vi "Signal processing testing.vi"() -> ()   [LabVIEW 2020]
doc: "This example demonstrates how to read N channels of analog input from a LINX device."
uses:
  <vilib>/MakerHub/LINX/Public/Peripherals/Analog/Analog Read N Chans.vi
  <vilib>/MakerHub/LINX/Private/Local IO/LinxAnalogRead.vi
  <vilib>/MakerHub/LINX/Public/Utilities/Check Channel.vi
  <vilib>/MakerHub/LINX/Public/Utilities/Open Serial.vi
  <vilib>/MakerHub/LINX/Private/Utilties/Generate Error.vi
  <vilib>/Analysis/Matrix/Numeric/Conversions/Array To Matrix - RA.vi
  <vilib>/Utility/file.llb/Write Delimited Spreadsheet (DBL).vi
  <vilib>/MakerHub/LINX/LMH-LINX.lvlib
  <vilib>/Analysis/Matrix/NI_Matrix.lvlib
panel:
  in  "B 6":dbl
  in  "A 6":dbl
  out "Weight":dbl
  out "Voltage 3":dbl
  in  "Analog Port 6":dbl
  in  "B 5":dbl
  in  "A 5":dbl
  out "Pressure (PSI) 2":dbl
  out "Voltage 2":dbl
  in  "Analog Port 5":dbl
  in  "Input pressure (PSI)":dbl
  in  "B 4":dbl
  in  "A 4":dbl
  out "Pressure (PSI)":dbl
  out "Voltage":dbl
  in  "Analog Port 4":dbl
  in  "C 3":dbl
  in  "B 3":dbl
  in  "A 3":dbl
  out "Temperature (F) 3":dbl
  out "Temperature (C) 3":dbl
  out "Temperature (K) 3":dbl
  out "Resistance 3":dbl
  in  "Analog Port 3":dbl
  in  "C 2":dbl
  in  "B 2":dbl
  in  "A 2":dbl
  out "Temperature (F) 2":dbl
  out "Temperature (C) 2":dbl
  out "Temperature (K) 2":dbl
  out "Resistance 2":dbl
  in  "Analog Port 2":dbl
  in  "Input temp (C)":dbl
  in  "C":dbl
  in  "B":dbl
  in  "A":dbl
  out "Temperature (F)":dbl
  out "Temperature (C)":dbl
  out "Temperature (K)":dbl
  out "WRITING TO FILE":bool
  in  "?":bool
  out "error out":errorcluster
  out "Full filepath":string
  in  "Path":path
  in  "File extension":string
  in  "Filename":string
  out "Resistance":dbl
  in  "Analog Port":dbl
  out "Time Stamp":timestamp
  out "PT1 reading":dbl(graph)
  in  "Stop Button":bool
  out "Loop Rate (Hz)":u32
  in  "Serial Port":refnum<visa-resource-name>
  # "Thermistor Calibration Program\nThis program gathers data points necessary to calibrate an NTC 10K Thermistor.\n It also allows for the testing of found A, B, and C values via user input."
  # "TM1"
  # "PT1"
  # "TM2"
  # "TM3"
  # "PT2"
  # "LC1"
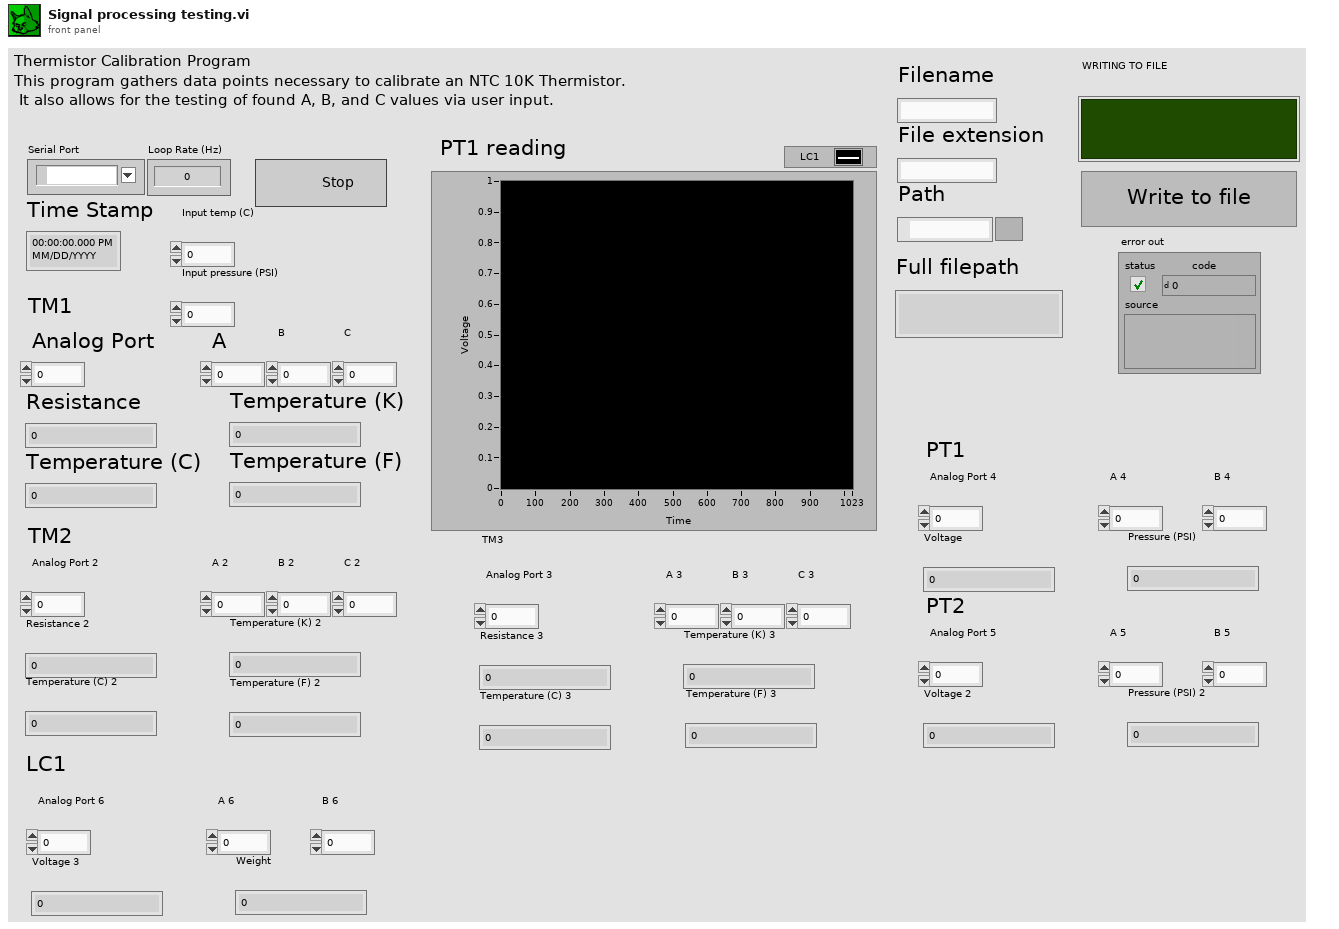
[diagram p1: front panel]
types:
  T1 = typedef "LMH-LINX.lvlib/LINX Ref.ctl" = cluster{"IO":T2, "Interface":T3, "LINX Device Config":T4}
  T2 = typedef "LMH-LINX.lvlib/Platform.ctl" = enum16{"Remote", "Local"}
  T3 = typedef "LMH-LINX.lvlib/Interface.ctl" = enum16{"Serial", "TCP"}
  T4 = typedef "LMH-LINX.lvlib/Device.lvlib/LINX Device Config.ctl" = cluster{"Interface":T3, "COM Port":refnum<visa-resource-name>, "TCP Configuration":T5, "Device Family":u8, "Device ID":u8, "Device Name":string, "TCP Ref":refnum<k5>, "Channels":T6}
  T5 = typedef "LMH-LINX.lvlib/Device.lvlib/TCP Config.ctl" = cluster{"IP Address":string, "Port":u16}
  T6 = typedef "LMH-LINX.lvlib/Channels.ctl" = cluster{"DI":u8[], "DO":u8[], "AI":u8[], "AO":u8[], "PWM":u8[], "QE":u8[], "UART":u8[], "I2C 2":u8[], "SPI":u8[], "CAN":u8[], "Servo":u8[], "AI Ref (V)":dbl, "AI Resolution (Bits)":u8, "AO Ref (V)":dbl, "AO Resolution (Bits)":u8}
  T7 = typedef "NI_Matrix.lvlib/RealMatrix.ctl" = dbl[][]
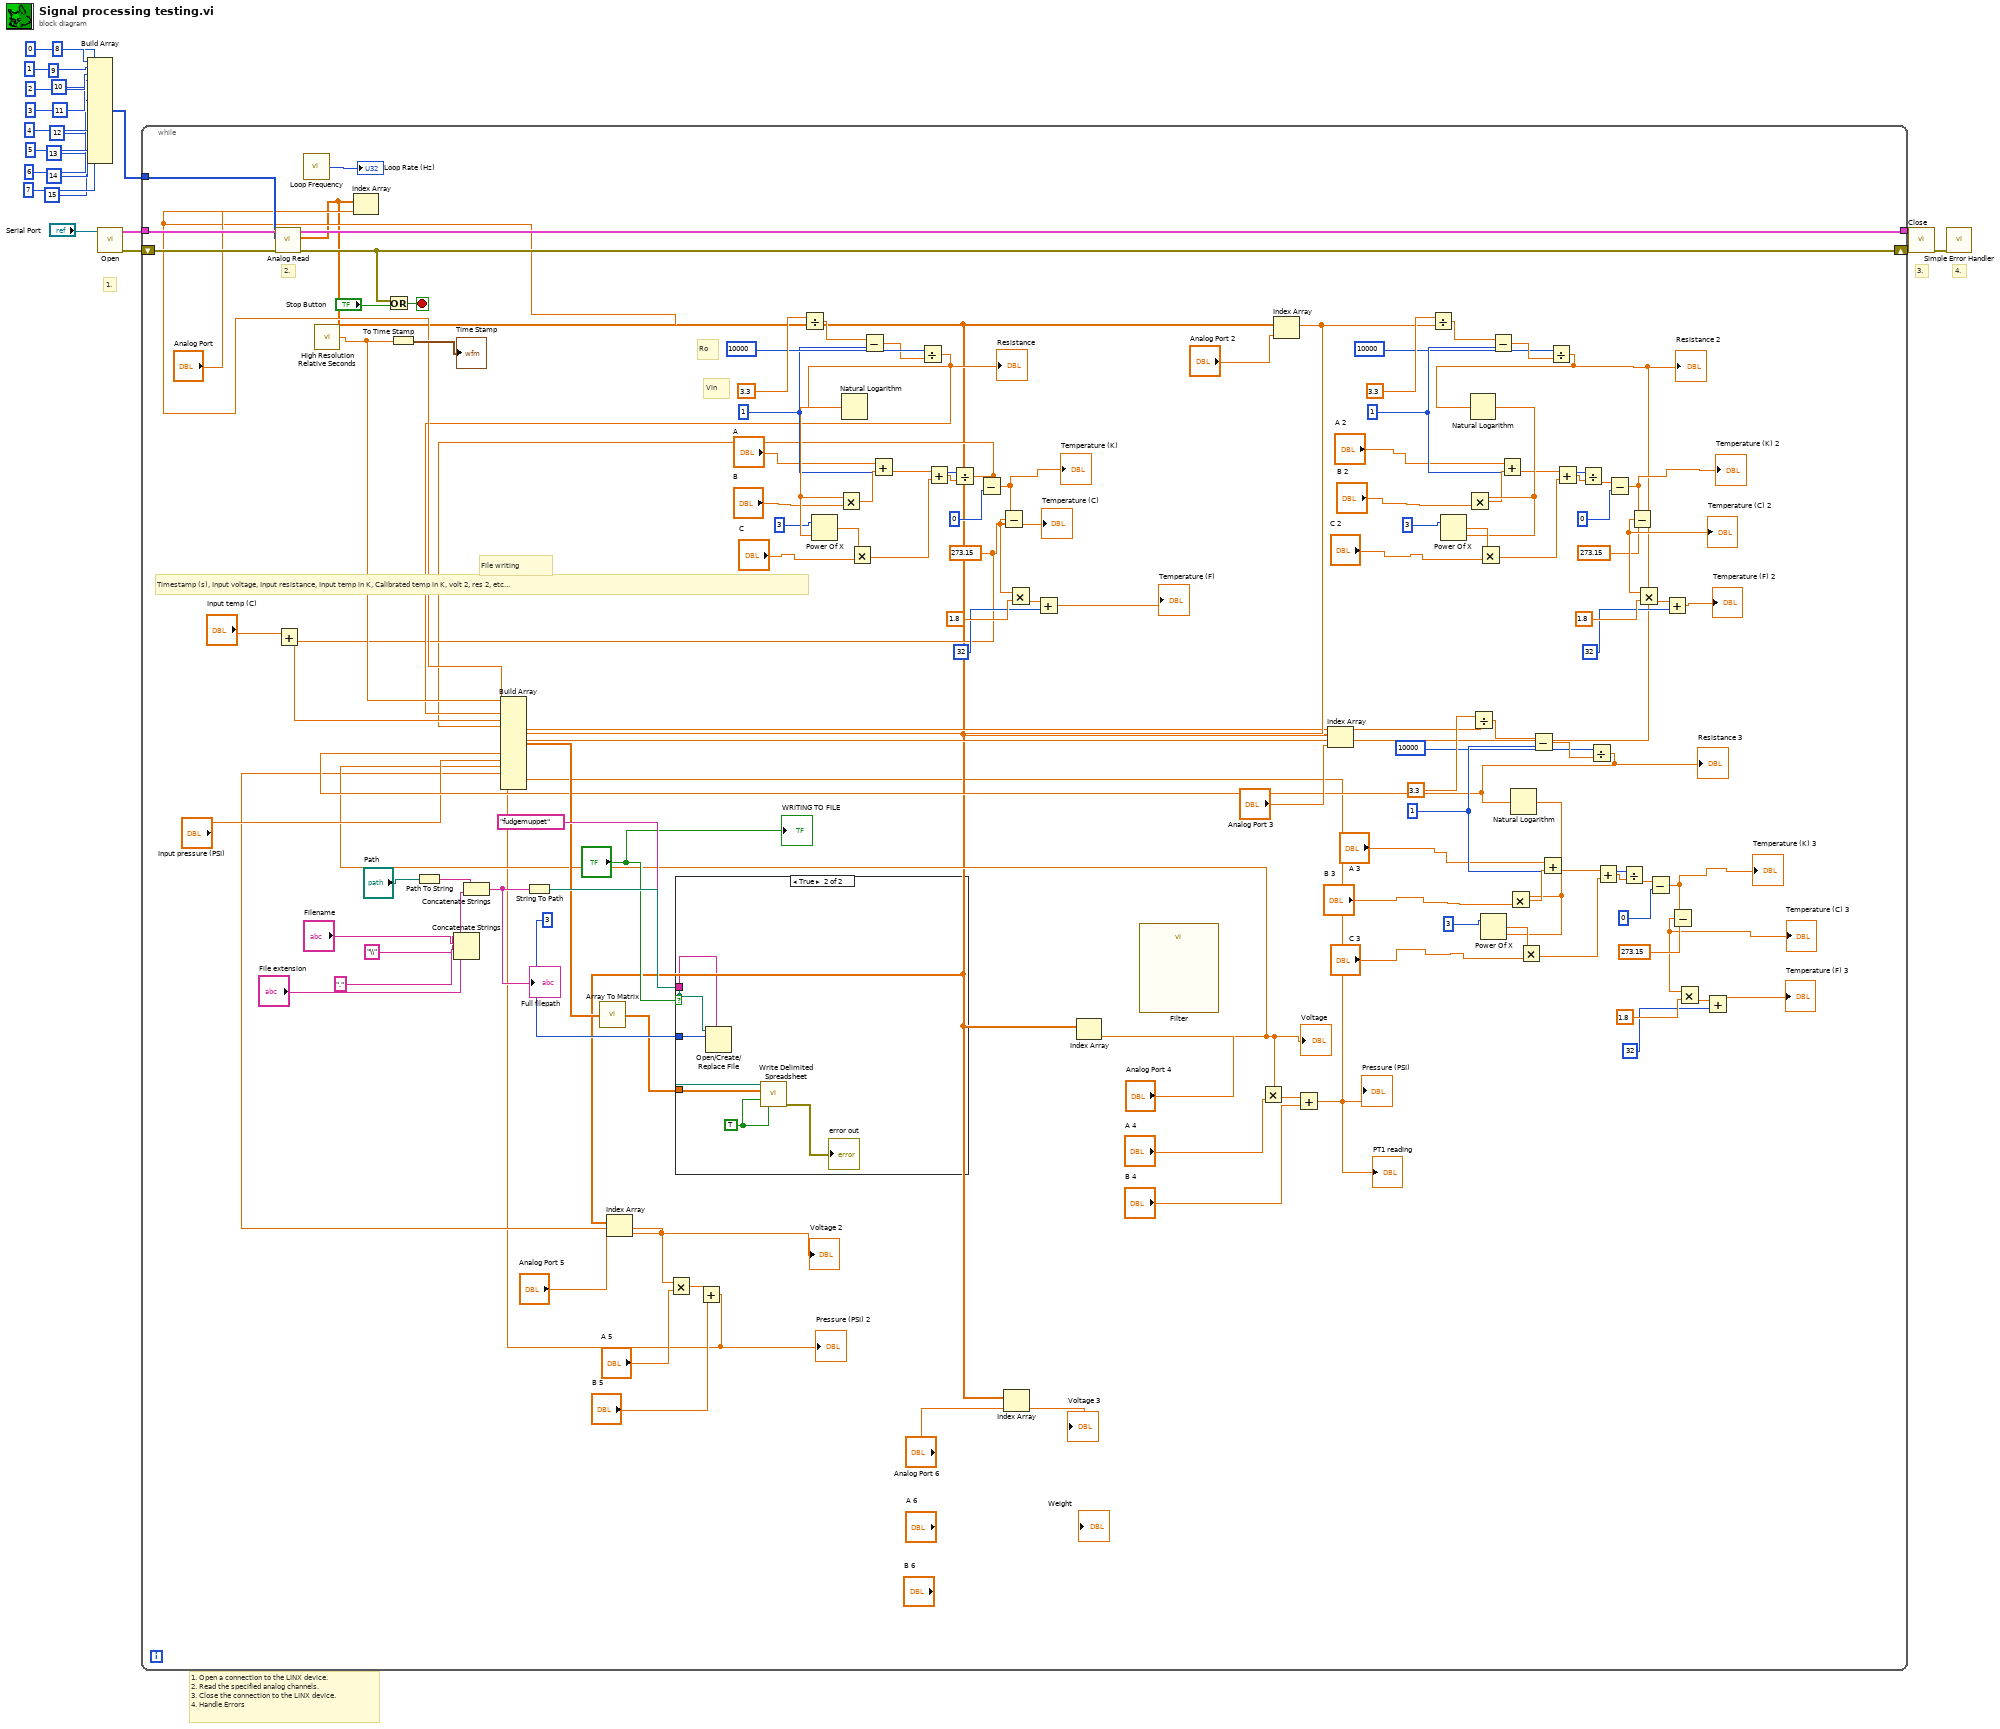
[diagram p0: block diagram]
diagram:
  # "1. Open a connection to the LINX device.\n2. Read the specified analog channels.\n3. Close the connection to the LINX device.\n4. Handle Errors"
  # "4."
  # "3."
  # "1."
  n1 = Build Array(0, 1, 2, 3, 4, 5, 6, 7, 8, 9, 10, 11, 12, 13, 14, 15) -> (w17:i32[])
  n2 = call-poly <vilib>:"Open.vi"("Serial Port"="Serial Port") -> ("Error Out"=w22:errorcluster, "LINX Resource"=w23:T1)  [unwired: 8 in, 1 out]
  n3 = while {
    tunnel: w23 -> [w146]
    tunnel: [w144] -> w21
    shift-right: [w141] -> w20
    shift-left: w22 -> [w145]
    tunnel: w17 -> [w140]
    stop <- w143 stop-if-true
    w61 = 1
    w84 = 1
    w100 = 273.15
    w109 = 1
    # "Timestamp (s), Input voltage, Input resistance, Input temp in K, Calibrated temp in K, volt 2, res 2, etc..."
    # "File writing"
    # "Vin"
    # "Ro"
    # "2."
    n4 = call-poly <vilib>:"Analog Read.vi"("Error In"=w145, "AI Channel(s)"=w140, "LINX Resource"=w146) -> ("Error Out"=w141:errorcluster, "Voltages"=w28:dbl[], "LINX Resource"=w144:T1)  [unwired: 5 in, 1 out]
    n5 = Add(x="Input temp (C)", y=w100) -> (x+y=w98:dbl)
    n6 = call <vilib>:"Loop Frequency.vi"() -> ("Loop Rate (Hz)"=→"Loop Rate (Hz)":u32)
    n7 = call <vilib>:"High Resolution Relative Seconds.vi"() -> ("relative seconds"=w122:dbl)
    n8 = Index Array(array=w28, index="Analog Port") -> (element=w120:dbl)
    n9 = Or(x=w141, y="Stop Button") -> (x .or. y?=w143:bool)
    n10 = To Time Stamp(1:w122) -> (0:→"Time Stamp":timestamp)
    n11 = Path To String(path="Path") -> (string=w135:string)
    n12 = Concatenate Strings("\\", "Filename", ".", "File extension") -> (w134:string)
    n13 = Concatenate Strings(w135, w134) -> (w133:string)
    "Full filepath" <- w133
    n14 = String To Path(string=w133) -> (path=w128:path)
    n15 = Index Array(array=w28, index="Analog Port 5") -> (element=w29:dbl)
    "Voltage 2" <- w29
    n16 = Multiply(x=w29, y="A 5") -> (x*y=w32:dbl)
    n17 = Add(x=w32, y="B 5") -> (x+y=w25:dbl)
    "Pressure (PSI) 2" <- w25
    n18 = Divide(x=3.3, y=w120) -> (x/y=w119:dbl)
    n19 = Subtract(x=w119, y=w109) -> (x-y=w117:dbl)
    n20 = Divide(x=10000, y=w117) -> (x/y=w101:dbl)
    "Resistance" <- w101
    n21 = Natural Logarithm(1:w101) -> (0:w115:dbl)
    n22 = Power Of X(1:w115, 2:3) -> (0:w116:dbl)
    n23 = Multiply(x=w115, y="B") -> (x*y=w112:dbl)
    n24 = Multiply(x=w116, y="C") -> (x*y=w111:dbl)
    n25 = Add(x="A", y=w112) -> (x+y=w113:dbl)
    n26 = Add(x=w113, y=w111) -> (x+y=w110:dbl)
    n27 = Divide(x=w109, y=w110) -> (x/y=w96:dbl)
    n28 = Subtract(x=w96, y=0) -> (x-y=w97:dbl)
    "Temperature (K)" <- w97
    n29 = Subtract(x=w97, y=w100) -> (x-y=w108:dbl)
    "Temperature (C)" <- w108
    n30 = Index Array(array=w28, index="Analog Port 6") -> (element=→"Voltage 3":dbl)
    n31 = Multiply(x=w108, y=1.8) -> (x*y=w106:dbl)
    n32 = Add(x=w106, y=32) -> (x+y=→"Temperature (F)":dbl)
    n33 = Index Array(array=w28, index="Analog Port 4") -> (element=w34:dbl)
    "Voltage" <- w34
    n34 = call "Filter"() -> ()  [unwired: 10 in, 2 out]
    n35 = Multiply(x=w34, y="A 4") -> (x*y=w37:dbl)
    n36 = Index Array(array=w28, index="Analog Port 2") -> (element=w46:dbl)
    n37 = Add(x=w37, y="B 4") -> (x+y=w24:dbl)
    "PT1 reading" <- w24
    "Pressure (PSI)" <- w24
    n38 = Index Array(array=w28, index="Analog Port 3") -> (element=w44:dbl)
    n39 = Divide(x=3.3, y=w46) -> (x/y=w93:dbl)
    n40 = Divide(x=3.3, y=w44) -> (x/y=w69:dbl)
    n41 = Subtract(x=w93, y=w84) -> (x-y=w92:dbl)
    n42 = Subtract(x=w69, y=w61) -> (x-y=w68:dbl)
    n43 = Divide(x=10000, y=w92) -> (x/y=w45:dbl)
    "Resistance 2" <- w45
    n44 = Natural Logarithm(1:w45) -> (0:w90:dbl)
    n45 = Power Of X(1:w90, 2:3) -> (0:w91:dbl)
    n46 = Multiply(x=w90, y="B 2") -> (x*y=w87:dbl)
    n47 = Multiply(x=w91, y="C 2") -> (x*y=w86:dbl)
    n48 = Add(x="A 2", y=w87) -> (x+y=w88:dbl)
    n49 = Add(x=w88, y=w86) -> (x+y=w85:dbl)
    n50 = Divide(x=w84, y=w85) -> (x/y=w80:dbl)
    n51 = Divide(x=10000, y=w68) -> (x/y=w43:dbl)
    "Resistance 3" <- w43
    n52 = Build Array(w122, w120, w101, w98, w96, w46, w45, w44, w43, "Input pressure (PSI)", w34, w29, w24, w25) -> (w123:dbl[])
    n53 = call-poly <vilib>:"Array To Matrix.vi"("Real 1D Array"=w123) -> ("Real Matrix (Column Vector)"=w124:T7)
    n54 = case shown="True" "?" {
      tunnel: w128 -> [_ w150]
      tunnel: w124 -> [_ w147]
      tunnel: "fudgemuppet" -> [_ w152]
      tunnel: 3 -> [_ w151]
      frame False {
      }
      frame True {
        w148 = TRUE
        n55 = Open/Create/Replace File(file path (use dialog)=w150, prompt=w152, operation (0:open)=w151) -> ()  [unwired: 3 in, 3 out]
        n56 = call-poly <vilib>:"Write Delimited Spreadsheet.vi"("file path (dialog if empty)"=w150, "2D data"=w147, "append to file? (new file:F)"=w148, "transpose? (no:F)"=w148) -> ("error out"=→"error out":errorcluster)  [unwired: 10 in, 1 out]
      }
    }
    n57 = Natural Logarithm(1:w43) -> (0:w53:dbl)
    n58 = Power Of X(1:w53, 2:3) -> (0:w67:dbl)
    n59 = Multiply(x=w53, y="B 3") -> (x*y=w64:dbl)
    n60 = Multiply(x=w67, y="C 3") -> (x*y=w63:dbl)
    n61 = Add(x="A 3", y=w64) -> (x+y=w65:dbl)
    n62 = Add(x=w65, y=w63) -> (x+y=w62:dbl)
    n63 = Subtract(x=w80, y=0) -> (x-y=w73:dbl)
    "Temperature (K) 2" <- w73
    n64 = Divide(x=w61, y=w62) -> (x/y=w57:dbl)
    n65 = Subtract(x=w73, y=273.15) -> (x-y=w72:dbl)
    "Temperature (C) 2" <- w72
    n66 = Multiply(x=w72, y=1.8) -> (x*y=w82:dbl)
    n67 = Subtract(x=w57, y=0) -> (x-y=w51:dbl)
    "Temperature (K) 3" <- w51
    n68 = Add(x=w82, y=32) -> (x+y=→"Temperature (F) 2":dbl)
    n69 = Subtract(x=w51, y=273.15) -> (x-y=w50:dbl)
    "Temperature (C) 3" <- w50
    n70 = Multiply(x=w50, y=1.8) -> (x*y=w59:dbl)
    n71 = Add(x=w59, y=32) -> (x+y=→"Temperature (F) 3":dbl)
    "WRITING TO FILE" <- "?"
  }
  n72 = call <vilib>:"Close.vi"("Error In"=w20, "LINX Resource"=w21) -> ("Error Out"=w18:errorcluster)  [unwired: 9 in]
  n73 = call <vilib>:"Simple Error Handler.vi"("error in (no error)"=w18) -> ()  [unwired: 4 in, 5 out]
